vi "Autonomous Independent.vi"   [LabVIEW 2017]
doc: "This VI is called when autonomous begins, and will automatically be terminated when autonomous ends. You can carry out timed or sensor driven robot movement independently without needing to return to the caller."
uses:
  <vilib>/Rock Robotics/WPI/Solenoid/WPI_SolenoidValue.ctl
  <vilib>/Rock Robotics/WPI/ThirdParty/Phoenix-LabVIEW/Motor Controller/Controls/CTRE_Phoenix_MotorControl_ControlMode.ctl
  <vilib>/Rock Robotics/Network Tables/NT Read Number.vi
  <vilib>/Rock Robotics/Network Tables/NT Read String.vi
  <vilib>/Rock Robotics/WPI/Solenoid/WPI_SolenoidSetEnum.vi
panel:
  # "Be sure to right-click and choose Data Operations>>Make Current Value default if you want to save the array values with the VI"
types:
  T1 = enum16{"cross_baseline_short", "cross_baseline_long", "hot_from_middle", "if_hot_2_if_cold_1", "if_hot_1_if_cold_1", "put_in_exchange"}
  T2 = typedef "WPI_DriverStationAllianceInfo.ctl" = enum16{"Red", "Blue", "Invalid"}
  T3 = typedef "WPI_SolenoidValue.ctl" = enum16{"Off", "On", "Forward", "Reverse"}
  T4 = typedef "WPI_MotorControlDeviceRef.ctl" = cluster{"DeviceStatus":errorcluster, "Type":T5, "PWM":cluster{"PWM Channel":T6, "DeadBand":T7}, "CAN":cluster{"Device Number":u8, "SetOutput VI Ref":variant, "GetOutput VI Ref":variant, "Enable VI Ref":variant, "Disable VI Ref":variant, "Data":variant}, "Invert":bool, "DIO PWM":cluster{"PWM \"Enable\" Channel":T6, "DIOChannel":T8, "PWM Rate":dbl}}
  T5 = typedef "WPI_MotorControlType.ctl" = enum16{"PWM", "CAN", "DIO PWM"}
  T6 = typedef "FPGA_DIOPWMChannel.ctl" = enum8{"PWM 0", "PWM 1", "PWM 2", "PWM 3", "PWM 4", "PWM 5", "PWM 6", "PWM 7", "PWM 8", "PWM 9", "PWM MXP 0", "PWM MXP 1", "PWM MXP 2", "PWM MXP 3", "PWM MXP 4", "PWM MXP 5", "PWM MXP 6", "PWM MXP 7", "PWM MXP 8", "PWM MXP 9", "Invalid"}
  T7 = typedef "WPI_PWMDeadband.ctl" = cluster{"Name":string, "maxPositivePwm":i32, "minPositivePwm":i32, "centerPwm":i32, "maxNegativePwm":i32, "minNegativePwm":i32, "angularRange":u16}
  T8 = typedef "FPGA_DIOChannel.ctl" = enum8{"DIO 0", "DIO 1", "DIO 2", "DIO 3", "DIO 4", "DIO 5", "DIO 6", "DIO 7", "DIO 8", "DIO 9", "DIO MXP 0", "DIO MXP 1", "DIO MXP 2", "DIO MXP 3", "DIO MXP 4", "DIO MXP 5", "DIO MXP 6", "DIO MXP 7", "DIO MXP 8", "DIO MXP 9", "DIO MXP 10", "DIO MXP 11", "DIO MXP 12", "DIO MXP 13", "DIO MXP 14", "DIO MXP 15", "SPI Port CS1", "SPI Port CS2", "SPI Port CS3", "SPI Port MISO", "SPI Port MOSI", "Invalid"}
  T9 = typedef "WPI_SolenoidDevRef.ctl" = cluster{"DevStatus":errorcluster, "Pneumatics Control Module":u8, "Forward Solenoid Channel":T10, "Reverse Solenoid Channel":T10}
  T10 = typedef "WPI_SolenoidChannel.ctl" = enum8{"Solenoid 0", "Solenoid 1", "Solenoid 2", "Solenoid 3", "Solenoid 4", "Solenoid 5", "Solenoid 6", "Solenoid 7", "Invalid"}
  T11 = typedef "CTRE_Phoenix_MotorControl_ControlMode.ctl" = u16
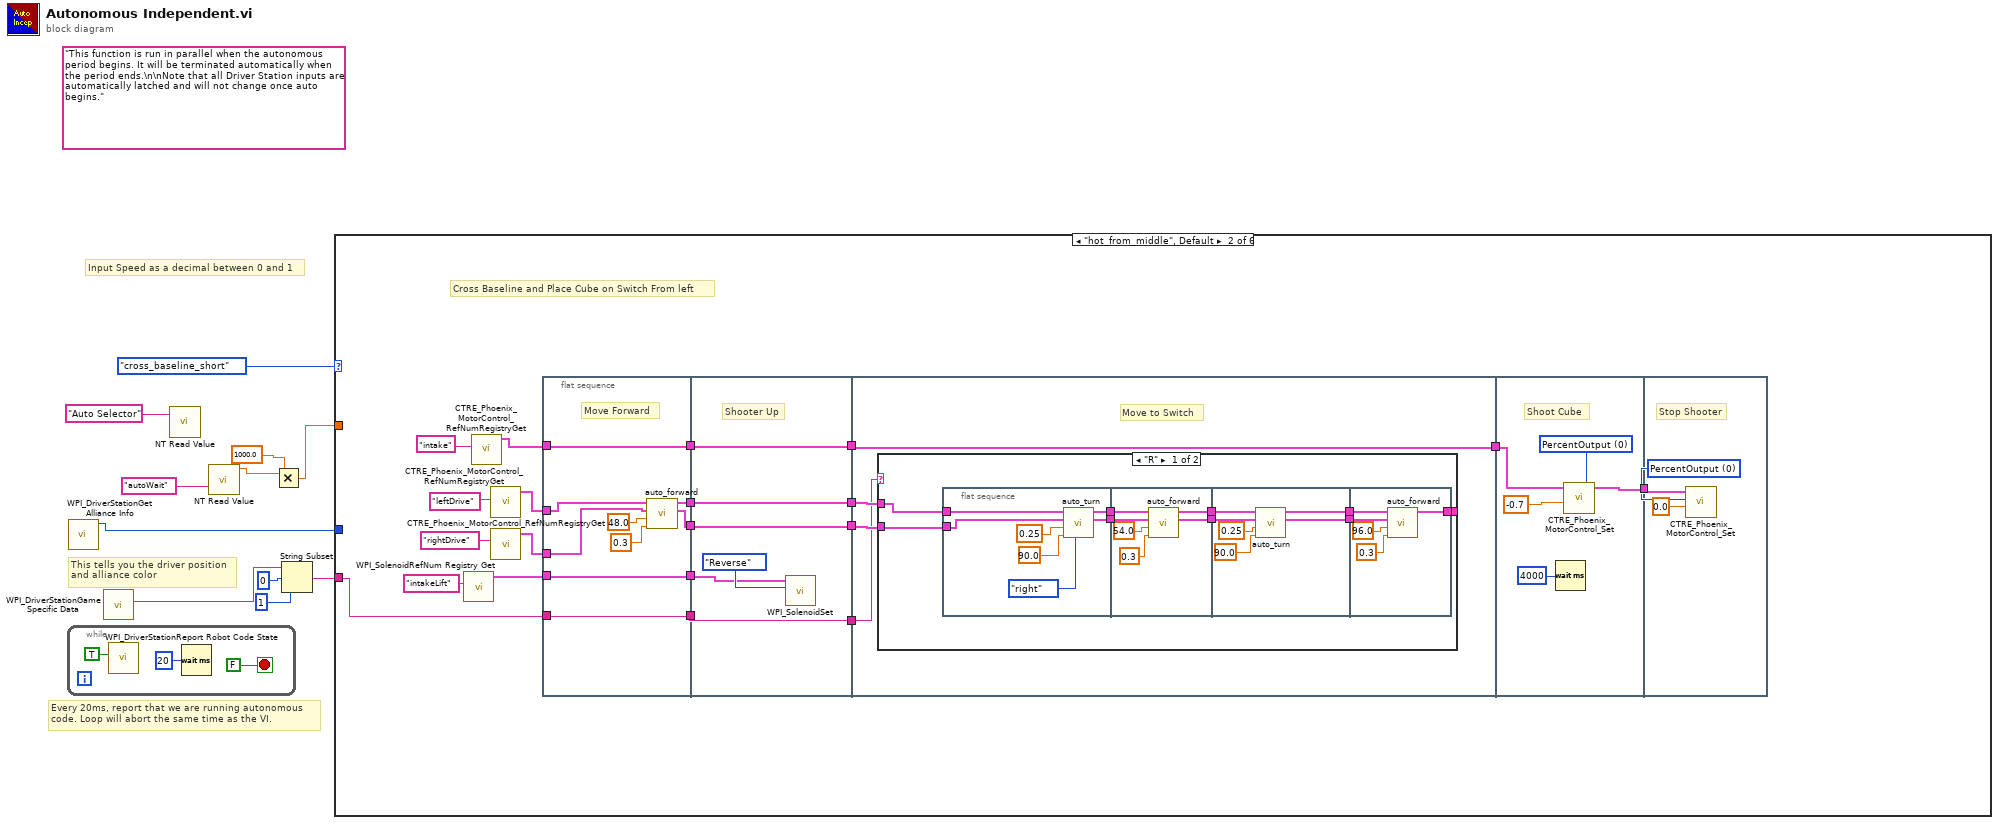
[diagram p0: block diagram]
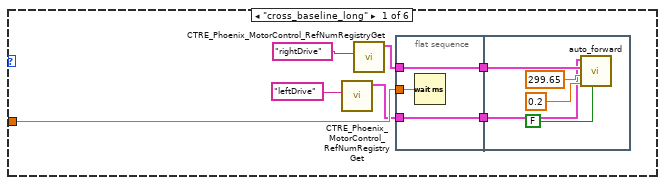
[diagram p2: hidden frame]
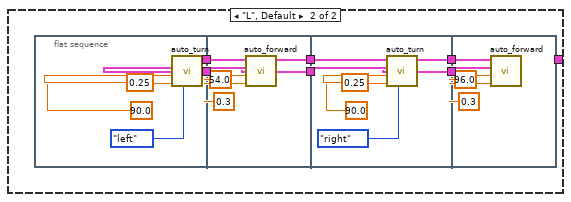
[diagram p3: hidden frame]
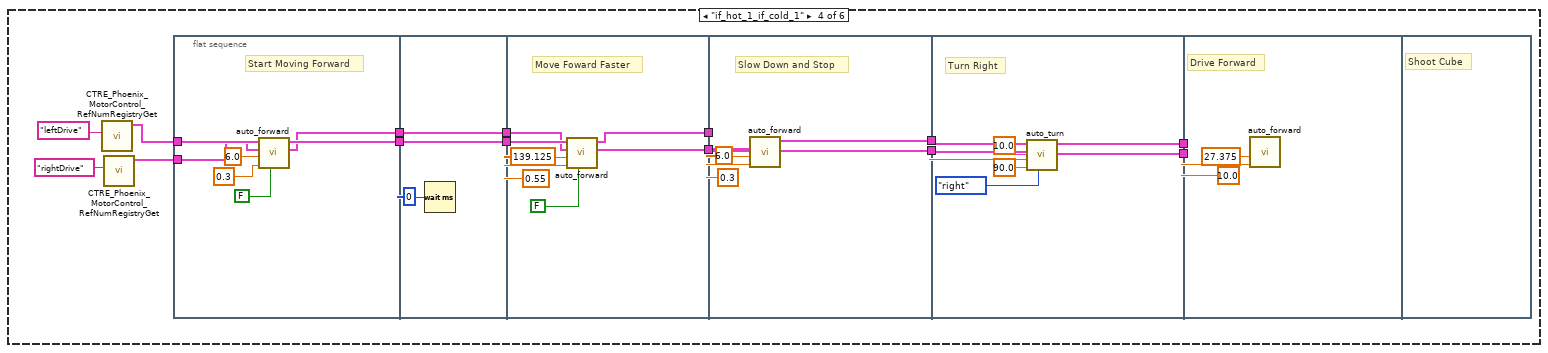
[diagram p5: hidden frame]
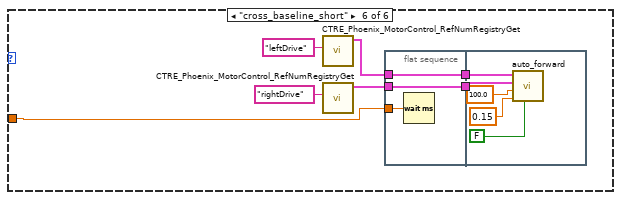
[diagram p7: hidden frame]
diagram:
  (unwired) "This function is run in parallel when the autonomous period begins. It will be terminated automatically when the period ends.\n\nNote that all Driver Station inputs are automatically latched and will not change once auto begins."
  # "Input Speed as a decimal between 0 and 1"
  # "Every 20ms, report that we are running autonomous\ncode. Loop will abort the same time as the VI."
  # "This tells you the driver position\nand alliance color"
  n1 = while {
    stop <- FALSE stop-if-true
    n2 = call <vilib>:"WPI_DriverStationReport Robot Code State.vi"("Autonomous"=TRUE) -> ()  [unwired: 10 in, 1 out]
    n3 = Wait (ms)(milliseconds to wait=u32 20) -> ()  [unwired: 1 out]
  }
  n4 = call <vilib>:"WPI_DriverStationGet Alliance Info.vi"() -> ("Alliance"=w11:T2)  [unwired: 11 out]
  n5 = call <vilib>:"WPI_DriverStationGame Specific Data.vi"() -> ("Game Specific Data"=w4:string)  [unwired: 11 in]
  n6 = call-poly <vilib>:"NT Read Value.vi"("Name"="Auto Selector") -> ()  [unwired: 9 in, 2 out]
  n7 = call-poly <vilib>:"NT Read Value.vi"("Name"="autoWait") -> ("Numeric"=w8:dbl)  [unwired: 9 in, 1 out]
  n8 = Multiply(x=w8, y=1000.0) -> (x*y=w6:dbl)
  n9 = String Subset(string=w4, offset (0)=0, length (rest)=1 ("length (rest)")) -> (substring=w1:string)
  n10 = case shown="\"hot_from_middle\", Default" T1."cross_baseline_short" {
    tunnel: w11 -> [_ _ _ _ _ _]
    tunnel: w6 -> [w21 _ _ _ _ w184]
    tunnel: w1 -> [_ w45 _ _ _ _]
    frame "cross_baseline_long" {
      n11 = call <vilib>:"CTRE_Phoenix_MotorControl_RefNumRegistryGet.vi"("refnum name"="leftDrive") -> ("PhoenixMotorControlDevRef"=w15:T4)  [unwired: 9 in, 1 out]
      n12 = call <vilib>:"CTRE_Phoenix_MotorControl_RefNumRegistryGet.vi"("refnum name"="rightDrive") -> ("PhoenixMotorControlDevRef"=w18:T4)  [unwired: 9 in, 1 out]
      n13 = flat-sequence {
        tunnel: w21 -> [w24]
        tunnel: [w23] -> w19
        tunnel: w18 -> [w23]
        tunnel: [w22] -> w16
        tunnel: w15 -> [w22]
        tunnel: w19 -> [w26]
        tunnel: w16 -> [w25]
        frame #0 {
          n14 = Wait (ms)(milliseconds to wait=w24) -> ()  [unwired: 1 out]
        }
        frame #1 {
          n15 = call "auto_forward.vi"("reverse?"=FALSE, "speed (decimal)"=0.2, "distance (in)"=299.65, "rightDrive"=w26, "leftDrive"=w25) -> ()  [unwired: 5 in, 2 out]
        }
      }
    }
    frame "hot_from_middle", Default {
      # "Cross Baseline and Place Cube on Switch From left"
      n16 = call <vilib>:"WPI_SolenoidRefNum Registry Get.vi"("refnum name"="intakeLift") -> ("SolenoidDevRef"=w42:T9)  [unwired: 9 in, 1 out]
      n17 = call <vilib>:"CTRE_Phoenix_MotorControl_RefNumRegistryGet.vi"("refnum name"="intake") -> ("PhoenixMotorControlDevRef"=w38:T4)  [unwired: 9 in, 1 out]
      n18 = call <vilib>:"CTRE_Phoenix_MotorControl_RefNumRegistryGet.vi"("refnum name"="leftDrive") -> ("PhoenixMotorControlDevRef"=w49:T4)  [unwired: 9 in, 1 out]
      n19 = call <vilib>:"CTRE_Phoenix_MotorControl_RefNumRegistryGet.vi"("refnum name"="rightDrive") -> ("PhoenixMotorControlDevRef"=w48:T4)  [unwired: 9 in, 1 out]
      n20 = flat-sequence {
        tunnel: w49 -> [w55]
        tunnel: w48 -> [w54]
        tunnel: w45 -> [w58]
        tunnel: [w58] -> w44
        tunnel: w42 -> [w56]
        tunnel: [w57] -> w39
        tunnel: w38 -> [w57]
        tunnel: [w56] -> w34
        tunnel: [w51] -> w32
        tunnel: [w50] -> w30
        tunnel: w44 -> [w63]
        tunnel: [w63] -> w43
        tunnel: w39 -> [w62]
        tunnel: [w62] -> w36
        tunnel: w34 -> [w61]
        tunnel: [w60] -> w33
        tunnel: w32 -> [w60]
        tunnel: [w59] -> w31
        tunnel: w30 -> [w59]
        tunnel: w43 -> [w65]
        tunnel: [w68] -> w37
        tunnel: w36 -> [w68]
        tunnel: w33 -> [w67]
        tunnel: w31 -> [w66]
        tunnel: w37 -> [w130]
        tunnel: [w132] -> w35
        tunnel: w35 -> [w137]
        frame #0 {
          # "Move Forward"
          n21 = call "auto_forward.vi"("speed (decimal)"=0.3, "distance (in)"=48.0, "rightDrive"=w54, "leftDrive"=w55) -> ("rightDrive"=w50:T4, "leftDrive"=w51:T4)  [unwired: 6 in]
        }
        frame #1 {
          # "Shooter Up"
          n22 = call-poly <vilib>:"WPI_SolenoidSet.vi"("Value"=WPI_SolenoidValue."Reverse", "SolenoidDevRef"=w61) -> ()  [unwired: 8 in, 2 out]
        }
        frame #2 {
          # "Move to Switch"
          n23 = case shown="\"R\"" w65 {
            tunnel: w67 -> [w77 _]
            tunnel: w66 -> [w76 _]
            tunnel: [w69 _] -> _
            frame "R" {
              n24 = flat-sequence {
                tunnel: w77 -> [w83]
                tunnel: w76 -> [w82]
                tunnel: [w79] -> w75
                tunnel: [w78] -> w74
                tunnel: w75 -> [w90]
                tunnel: w74 -> [w89]
                tunnel: [w86] -> w73
                tunnel: [w85] -> w72
                tunnel: w73 -> [w94]
                tunnel: w72 -> [w93]
                tunnel: [w92] -> w71
                tunnel: [w91] -> w70
                tunnel: w71 -> [w101]
                tunnel: w70 -> [w100]
                tunnel: [w97] -> w69
                frame #0 {
                  n25 = call "auto_turn.vi"("direction"=enum16{"right", "left"}."right", "angle"=90.0, "speed"=0.25, "rightDrive"=w82, "leftDrive"=w83) -> ("rightDrive"=w78:T4, "leftDrive"=w79:T4)  [unwired: 5 in]
                }
                frame #1 {
                  n26 = call "auto_forward.vi"("speed (decimal)"=0.3, "distance (in)"=54.0, "rightDrive"=w89, "leftDrive"=w90) -> ("rightDrive"=w85:T4, "leftDrive"=w86:T4)  [unwired: 6 in]
                }
                frame #2 {
                  n27 = call "auto_turn.vi"("angle"=90.0, "speed"=0.25, "rightDrive"=w93, "leftDrive"=w94) -> ("rightDrive"=w91:T4, "leftDrive"=w92:T4)  [unwired: 6 in]
                }
                frame #3 {
                  n28 = call "auto_forward.vi"("speed (decimal)"=0.3, "distance (in)"=96.0, "rightDrive"=w100, "leftDrive"=w101) -> ("leftDrive"=w97:T4)  [unwired: 6 in, 1 out]
                }
              }
            }
            frame "L", Default {
              n29 = flat-sequence {
                tunnel: [w109] -> w107
                tunnel: [w108] -> w106
                tunnel: w107 -> [w118]
                tunnel: w106 -> [w117]
                tunnel: [w114] -> w105
                tunnel: [w113] -> w104
                tunnel: w105 -> [w125]
                tunnel: w104 -> [w124]
                tunnel: [w120] -> w103
                tunnel: [w119] -> w102
                tunnel: w103 -> [w129]
                tunnel: w102 -> [w128]
                frame #0 {
                  n30 = call "auto_turn.vi"("direction"=enum16{"right", "left"}."left", "angle"=90.0, "speed"=0.25) -> ("rightDrive"=w108:T4, "leftDrive"=w109:T4)  [unwired: 7 in]
                }
                frame #1 {
                  n31 = call "auto_forward.vi"("speed (decimal)"=0.3, "distance (in)"=54.0, "rightDrive"=w117, "leftDrive"=w118) -> ("rightDrive"=w113:T4, "leftDrive"=w114:T4)  [unwired: 6 in]
                }
                frame #2 {
                  n32 = call "auto_turn.vi"("direction"=enum16{"right", "left"}."right", "angle"=90.0, "speed"=0.25, "rightDrive"=w124, "leftDrive"=w125) -> ("rightDrive"=w119:T4, "leftDrive"=w120:T4)  [unwired: 5 in]
                }
                frame #3 {
                  n33 = call "auto_forward.vi"("speed (decimal)"=0.3, "distance (in)"=96.0, "rightDrive"=w128, "leftDrive"=w129) -> ()  [unwired: 6 in, 2 out]
                }
              }
            }
          }
        }
        frame #3 {
          w131 = T11 0 items=["PercentOutput"=0, "Position"=1, "Velocity"=2, "Current"=3, "Follower"=5, "MotionProfile"=6, "MotionMagic"=7, "MotionMagicArc"=8, "MotionProfileArc"=10, "Disabled"=15] ("Control Mode")
          # "Shoot Cube"
          n34 = Wait (ms)(milliseconds to wait=u32 4000) -> ()  [unwired: 1 out]
          n35 = call <vilib>:"CTRE_Phoenix_MotorControl_Set.vi"("Output"=-0.7, "Control Mode"=w131, "PhoenixMotorControlDevRef"=w130) -> ("PhoenixMotorControlDevRef"=w132:T4)  [unwired: 7 in, 1 out]
        }
        frame #4 {
          w136 = T11 0 items=["PercentOutput"=0, "Position"=1, "Velocity"=2, "Current"=3, "Follower"=5, "MotionProfile"=6, "MotionMagic"=7, "MotionMagicArc"=8, "MotionProfileArc"=10, "Disabled"=15] ("Control Mode")
          # "Stop Shooter"
          n36 = call <vilib>:"CTRE_Phoenix_MotorControl_Set.vi"("Output"=0.0, "Control Mode"=w136, "PhoenixMotorControlDevRef"=w137) -> ()  [unwired: 7 in, 2 out]
        }
      }
    }
    frame "if_hot_2_if_cold_1" {
    }
    frame "if_hot_1_if_cold_1" {
      n37 = call <vilib>:"CTRE_Phoenix_MotorControl_RefNumRegistryGet.vi"("refnum name"="leftDrive") -> ("PhoenixMotorControlDevRef"=w141:T4)  [unwired: 9 in, 1 out]
      n38 = call <vilib>:"CTRE_Phoenix_MotorControl_RefNumRegistryGet.vi"("refnum name"="rightDrive") -> ("PhoenixMotorControlDevRef"=w140:T4)  [unwired: 9 in, 1 out]
      n39 = flat-sequence {
        tunnel: [w155] -> w144
        tunnel: [w154] -> w142
        tunnel: w141 -> [w153]
        tunnel: w140 -> [w152]
        tunnel: [w160] -> w145
        tunnel: w144 -> [w160]
        tunnel: [w159] -> w143
        tunnel: w142 -> [w159]
        tunnel: [w166] -> w151
        tunnel: [w165] -> w150
        tunnel: w145 -> [w163]
        tunnel: w143 -> [w162]
        tunnel: w151 -> [_]
        tunnel: [w170] -> w149
        tunnel: w150 -> [_]
        tunnel: [w169] -> w148
        tunnel: w149 -> [w178]
        tunnel: w148 -> [w177]
        tunnel: [w174] -> w147
        tunnel: [w173] -> w146
        tunnel: w147 -> [_]
        tunnel: w146 -> [_]
        frame #0 {
          # "Start Moving Forward"
          n40 = call "auto_forward.vi"("reverse?"=FALSE, "speed (decimal)"=0.3 ("speed (%)"), "distance (in)"=6.0, "rightDrive"=w152, "leftDrive"=w153) -> ("rightDrive"=w154:T4, "leftDrive"=w155:T4)  [unwired: 5 in]
        }
        frame #1 {
          n41 = Wait (ms)(milliseconds to wait=u32 0) -> ()  [unwired: 1 out]
        }
        frame #2 {
          # "Move Foward Faster"
          n42 = call "auto_forward.vi"("reverse?"=FALSE, "speed (decimal)"=0.55 ("speed (%)"), "distance (in)"=139.125, "rightDrive"=w162, "leftDrive"=w163) -> ("rightDrive"=w165:T4, "leftDrive"=w166:T4)  [unwired: 5 in]
        }
        frame #3 {
          # "Slow Down and Stop"
          n43 = call "auto_forward.vi"("speed (decimal)"=0.3 ("speed (%)"), "distance (in)"=6.0) -> ("rightDrive"=w169:T4, "leftDrive"=w170:T4)  [unwired: 8 in]
        }
        frame #4 {
          # "Turn Right"
          n44 = call "auto_turn.vi"("direction"=enum16{"right", "left"}."right", "angle"=90.0, "speed"=10.0, "rightDrive"=w177, "leftDrive"=w178) -> ("rightDrive"=w173:T4, "leftDrive"=w174:T4)  [unwired: 5 in]
        }
        frame #5 {
          # "Drive Forward"
          n45 = call "auto_forward.vi"("speed (decimal)"=10.0 ("speed (%)"), "distance (in)"=27.375) -> ()  [unwired: 8 in, 2 out]
        }
        frame #6 {
          # "Shoot Cube"
        }
      }
    }
    frame "put_in_exchange" {
    }
    frame "cross_baseline_short" {
      n46 = call <vilib>:"CTRE_Phoenix_MotorControl_RefNumRegistryGet.vi"("refnum name"="leftDrive") -> ("PhoenixMotorControlDevRef"=w188:T4)  [unwired: 9 in, 1 out]
      n47 = call <vilib>:"CTRE_Phoenix_MotorControl_RefNumRegistryGet.vi"("refnum name"="rightDrive") -> ("PhoenixMotorControlDevRef"=w185:T4)  [unwired: 9 in, 1 out]
      n48 = flat-sequence {
        tunnel: w184 -> [w191]
        tunnel: w188 -> [w190]
        tunnel: [w190] -> w187
        tunnel: [w189] -> w186
        tunnel: w185 -> [w189]
        tunnel: w187 -> [w193]
        tunnel: w186 -> [w192]
        frame #0 {
          n49 = Wait (ms)(milliseconds to wait=w191) -> ()  [unwired: 1 out]
        }
        frame #1 {
          n50 = call "auto_forward.vi"("reverse?"=FALSE, "speed (decimal)"=0.15, "distance (in)"=100.0, "rightDrive"=w192, "leftDrive"=w193) -> ()  [unwired: 5 in, 2 out]
        }
      }
    }
  }
